vi "GyroReset.vi"() -> (0 "Heading":dbl)   [LabVIEW 2017, in "DriveAuto.lvclass"]
uses:
  DriveAuto.lvclass
  Team-code/SensorDataGlobal.vi
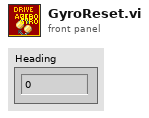
[diagram p1: front panel]
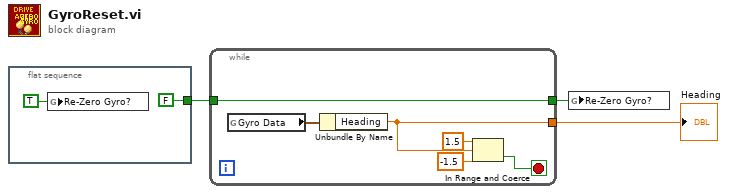
[diagram p0: block diagram]
diagram:
  n1 = flat-sequence {
    tunnel: [FALSE ("Re-Zero Gyro?")] -> w3
    frame #0 {
      n2 = global write "SensorDataGlobal.vi" "Re-Zero Gyro?"(TRUE ("Re-Zero Gyro?")) -> ()
    }
  }
  n3 = while {
    tunnel: [w11] -> w2
    tunnel: w3 -> [w11]
    tunnel: [w9] -> w1
    stop <- w6 stop-if-true
    n4 = global read "SensorDataGlobal.vi" "Gyro Data"() -> (w10:cluster{"Heading":dbl, "Gyro Raw":dbl})
    n5 = Unbundle By Name(w10) -> ("Heading"=w9:dbl)
    n6 = In Range and Coerce(upper limit=1.5, x=w9, lower limit=-1.5) -> (In Range?=w6:bool)  [unwired: 1 out]
  }
  "Heading" <- w1
  n7 = global write "SensorDataGlobal.vi" "Re-Zero Gyro?"(w2) -> ()
